vi "turbine controller 130319.vi"() -> ()   [LabVIEW 2022 SP3]
uses:
  <vilib>/Instr/_visa.llb/VISA Configure Serial Port (Instr).vi
panel:
  in  "clear":bool
  out "Current":dbl(graph)=1045.25
  in  "Set speed (approx)":i32(slide) scale=0.0..4000.0
  in  "send":bool
  in  "stop":bool
  in  "VISA resource name":refnum<visa-resource-name>="COM22"
  # "Note: Speed and current measurements have not been calibrated yet. So do not take absolute values here as accurate. \n\nThey are however linear*, so the calibration can be done after data collection.  \n\n*Encoder speed against tachometer measurement and current against multimeter current measurement. \n\nGW Mar19"
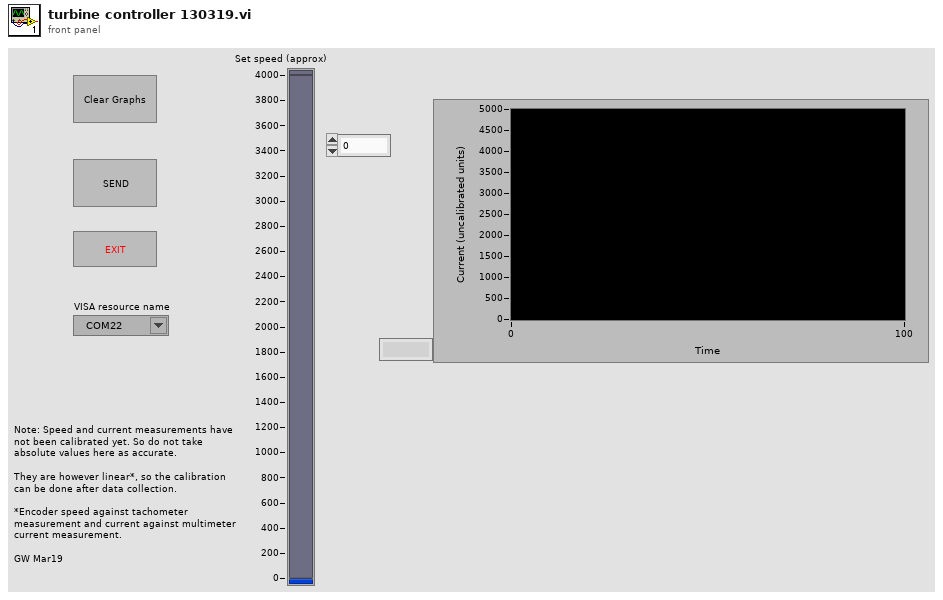
[diagram p1: front panel]
types:
  T1 = cluster{"baud rate":u32, "data bits":u16, "parity":enum16{"None", "Odd", "Even", "Mark", "Space"}, "stop bits":u16, "flow control":u16}
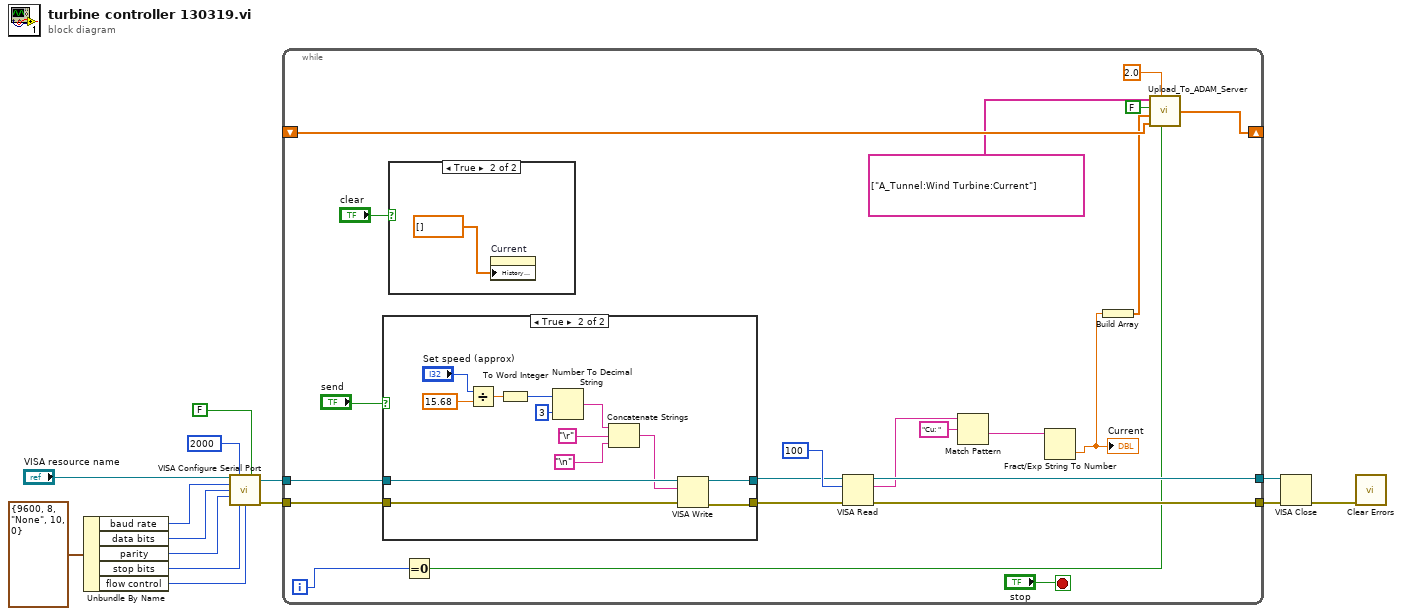
[diagram p0: block diagram]
diagram:
  n1 = Unbundle By Name(T1 {"baud rate"=9600, "data bits"=8, "parity"=enum."None", "stop bits"=10, "flow control"=0} ("Serial Settings")) -> ("baud rate"=w13:u32, "data bits"=w12:u16, "parity"=w11:enum16{"None", "Odd", "Even", "Mark", "Space"}, "stop bits"=w10:u16, "flow control"=w9:u16)
  n2 = call-poly "VISA Configure Serial Port"("VISA resource name"="VISA resource name", "timeout (10sec)"=u32 2000, "Enable Termination\nChar (T)"=FALSE ("Enable Termination\nChar (T)"), "baud rate (9600)"=w13, "data bits (8)"=w12, "parity (0:none)"=w11, "stop bits (10: 1 bit)"=w10, "flow control (0:none)"=w9) -> ("VISA resource name out"=w4:refnum<visa-resource-name>, "error out"=w5:errorcluster)  [unwired: 1 in, 5 out]
  n3 = while {
    tunnel: w5 -> [w36]
    tunnel: [w29] -> w3
    tunnel: [w30] -> w2
    tunnel: w4 -> [w35]
    shift-right: [w22] -> _
    shift-left: _ -> [w23]
    i -> [w17]
    stop <- "stop" stop-if-true
    n4 = case shown="True" "send" {
      tunnel: w36 -> [w38 w52]
      tunnel: [w39 w48] -> w32
      tunnel: w35 -> [w39 w51]
      tunnel: [w38 w47] -> w31
      frame False {
      }
      frame True {
        n5 = Divide(x="Set speed (approx)", y=15.68) -> (x/y=w41:dbl)
        n6 = To Word Integer(number=w41) -> (16bit integer=w40:i16)
        n7 = Number To Decimal String(number=w40, width (-)=i16 3) -> (decimal integer string=w46:string)
        n8 = Concatenate Strings(w46, "\r", "\n") -> (w44:string)
        n9 = VISA Write(VISA resource name=w51, write buffer=w44, error in (no error)=w52) -> (VISA resource name out=w48:refnum<visa-resource-name>, error out=w47:errorcluster)  [unwired: 1 out]
      }
    }
    n10 = case shown="True" "clear" {
      frame False {
      }
      frame True {
        n11 = property on="Current" class="WFChart (strict)"("History Data"=dbl[] []) -> ()  [unwired: 2 in, 2 out]
      }
    }
    n12 = Equal To 0?(x=w17) -> (x = 0?=w16:bool)
    n13 = VISA Read(VISA resource name=w32, byte count=u32 100, error in (no error)=w31) -> (VISA resource name out=w30:refnum<visa-resource-name>, read buffer=w27:string, error out=w29:errorcluster)  [unwired: 1 out]
    n14 = Match Pattern(string=w27, regular expression="Cu: ") -> (after substring=w26:string)  [unwired: 1 in, 3 out]
    n15 = Fract/Exp String To Number(string=w26) -> (number=w21:dbl)  [unwired: 3 in, 1 out]
    "Current" <- w21
    n16 = Build Array(w21) -> (w20:dbl[])
    n17 = call "Upload_To_ADAM_Server.vi"("First Loop"=w16, "Averaging Period (s)"=2.0, "Shift In"=w23, "Channel Values"=w20, "Give Variance"=FALSE, "Channel Names"=string[] ["A_Tunnel:Wind Turbine:Current"]) -> ("Shift Out"=w22:dbl[])
  }
  n18 = VISA Close(VISA resource name=w2, error in (no error)=w3) -> (error out=w1:errorcluster)
  n19 = call <vilib>:"Clear Errors.vi"("error in (no error)"=w1) -> ()  [unwired: 5 in, 2 out]
